vi "packageTelemetrySnapshot.vi"(8 "Error In":errorcluster, 10 "All Data":T2 {"Power Readings"."Current" format="%#.3g A"; "Power Readings"."Power" format="%#.3g W"; "Power Readings"."Shunt Voltage" format=" %#.3g V"; "Power Readings"."Bus Voltage" format="%#.3g V"; "Power Readings"."Voltage (Total)" format="%#.3g V"; "ThermalReadings"."Ambient Temp (°F)" format="%.2f °F"; "ThermalReadings"."Ambient Temp (°C)" format="%.2f °C"; "ThermalReadings"."Object Temp (°F)" format="%.2f °F"; "ThermalReadings"."Object Temp (°C)" format="%.2f °C"; "CPU loads"."ISR (%)" format="%#.2f"; "CPU loads"."Idle (%)" format="%#.2f"; "CPU loads"."Background (%)" format="%#.2f"; "CPU loads"."Normal (%)" format="%#.2f"; "CPU loads"."Above Normal (%)" format="%#.2f"; "CPU loads"."High (%)" format="%#.2f"; "CPU loads"."Timed Structures (%)" format="%#.2f"; "CPU loads"."Time Critical (%)" format="%#.2f"; "CPU loads"."Total (%)" format="%#.2f"}, 11 "Send Non-Critical Data":bool) -> (0 "Error Out":errorcluster, 2 "Pod Health":T1, 3 "Latest Critical Telemetry":T12)   [LabVIEW 2018]
uses:
  Type Defs/PodState.ctl
  Type Defs/criticalTelemetry.ctl
  Type Defs/prettyTelemetry.ctl
  Type Defs/ThermalReadings.ctl
  Type Defs/PodHealthConfig.ctl
  Sensors/Power Sensor - Adafruit INA219/INA219 Measurements.ctl
  Type Defs/tempReadings.ctl
  Type Defs/AnalogPressureReading.ctl
  Type Defs/allLaserReadings.ctl
  Type Defs/tofReading.ctl
  <vilib>/Utility/RT CPU Load.ctl
  Type Defs/pressureReading.ctl
  Type Defs/allData.ctl
  Type Defs/laserReading.ctl
  Type Defs/PodHealth.ctl
panel:
  out "UDP Data Packet":string
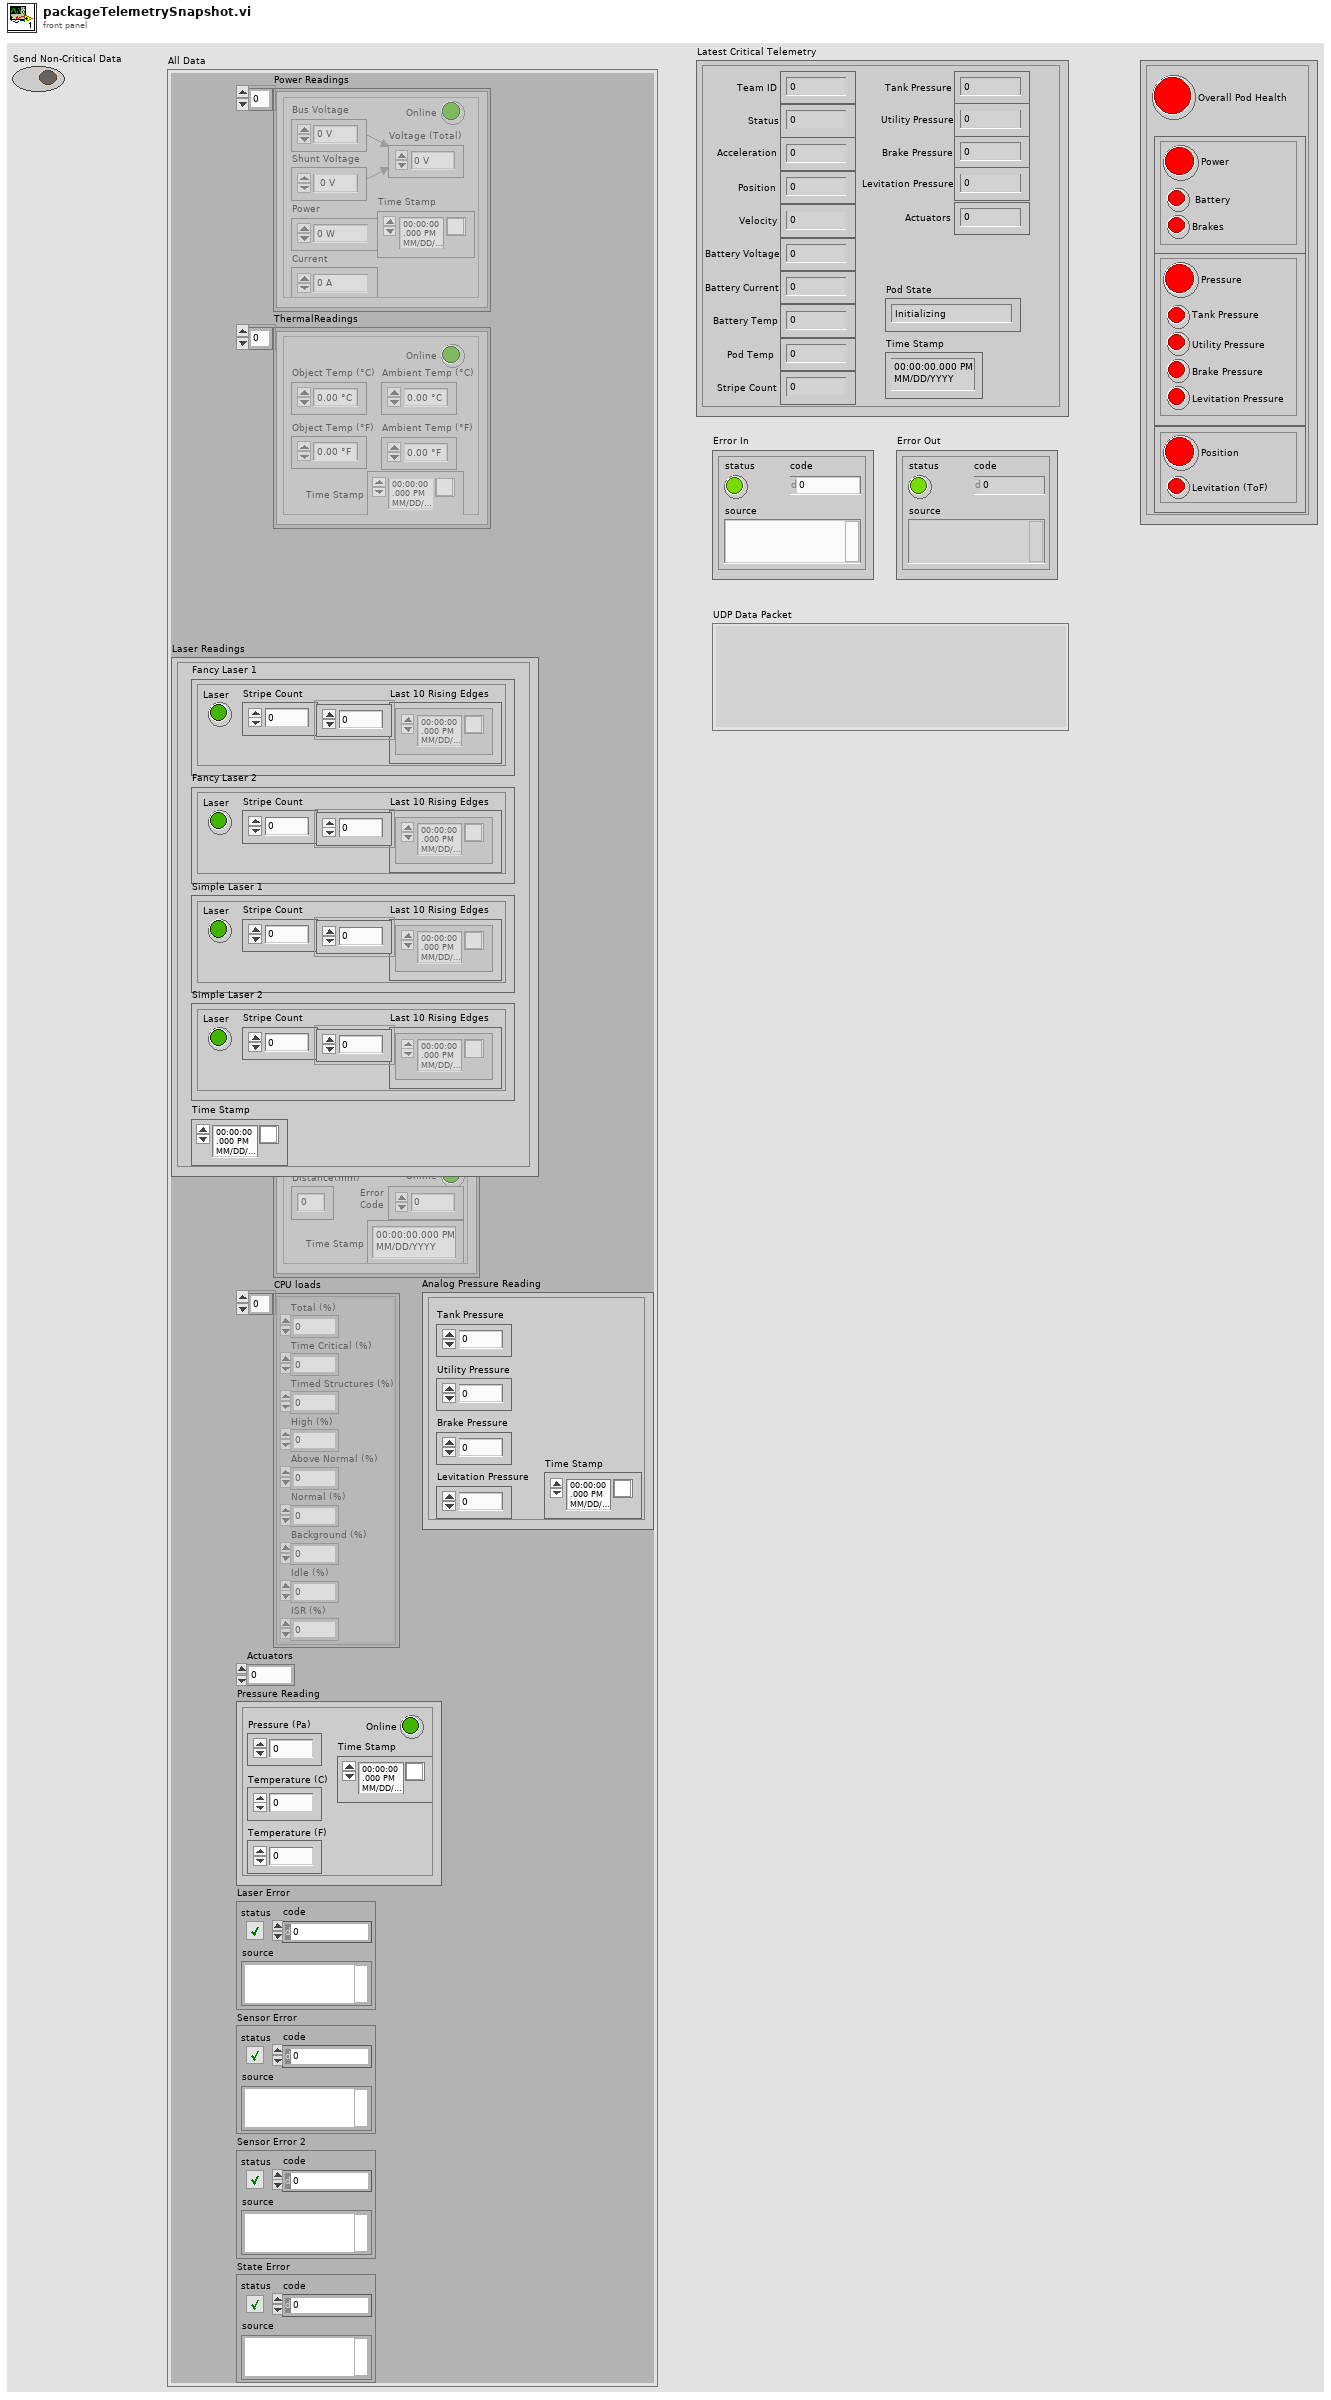
[diagram p1: front panel]
types:
  T1 = typedef "PodHealth.ctl" = cluster{"Overall Pod Health":bool, "Power":cluster{"Power":bool, " Battery":bool, "Brakes":bool}, "Pressure":cluster{"Pressure":bool, "Tank Pressure":bool, "Utility Pressure":bool, "Brake Pressure":bool, "Levitation Pressure":bool}, "Position":cluster{"Position":bool, "Levitation (ToF)":bool}}
  T2 = typedef "allData.ctl" = cluster{"Power Readings":T3[], "ThermalReadings":T4[], "Analog Pressure Reading":T5, "Laser Readings":T6, "Pod State":T8, "seconds since 1Jan1904":timestamp, "ToF Readings":T9[], "CPU loads":T10[], "Actuators":u32, "Pressure Reading":T11, "Laser Error":errorcluster, "Sensor Error":errorcluster, "Sensor Error 2":errorcluster, "State Error":errorcluster}
  T3 = typedef "INA219 Measurements.ctl" = cluster{"Voltage (Total)":dbl, "Bus Voltage":dbl, "Shunt Voltage":dbl, "Power":dbl, "Current":dbl, "Online":bool, "Time Stamp":timestamp}
  T4 = typedef "tempReadings.ctl" = cluster{"Object Temp (°C)":dbl, "Object Temp (°F)":dbl, "Ambient Temp (°C)":dbl, "Ambient Temp (°F)":dbl, "Online":bool, "Time Stamp":timestamp}
  T5 = typedef "AnalogPressureReading.ctl" = cluster{"Tank Pressure":dbl, "Utility Pressure":dbl, "Brake Pressure":dbl, "Levitation Pressure":dbl, "Time Stamp":timestamp}
  T6 = typedef "allLaserReadings.ctl" = cluster{"Fancy Laser 1":T7, "Fancy Laser 2":T7, "Simple Laser 1":T7, "Simple Laser 2":T7, "Time Stamp":timestamp}
  T7 = typedef "laserReading.ctl" = cluster{"Laser":bool, "Stripe Count":u32, "Last 10 Rising Edges":timestamp[]}
  T8 = typedef "PodState.ctl" = enum16{"Initializing", "Pre-flight Testing", "Ready", "Pushing", "Coast", "Braking", "Pod-Stop", "Fault"}
  T9 = typedef "tofReading.ctl" = cluster{"Distance(mm)":u8, "Online":bool, "Error\nCode":u8, "Time Stamp":timestamp}
  T10 = typedef "NI_Real-Time Target Support.lvlib/RT CPU Load.ctl" = cluster{"Total (%)":dbl, "Time Critical (%)":dbl, "Timed Structures (%)":dbl, "High (%)":dbl, "Above Normal (%)":dbl, "Normal (%)":dbl, "Background (%)":dbl, "Idle (%)":dbl, "ISR (%)":dbl}
  T11 = typedef "pressureReading.ctl" = cluster{"Time Stamp":timestamp, "Online":bool, "Temperature (C)":dbl, "Pressure (Pa)":dbl, "Temperature (F)":dbl}
  T12 = typedef "criticalTelemetry.ctl" = cluster{"Team ID":u8, "Status":u8, "Acceleration":dbl, "Position":dbl, "Velocity":dbl, "Battery Voltage":dbl, "Battery Current":dbl, "Battery Temp":dbl, "Pod Temp":dbl, "Stripe Count":u32, "Tank Pressure":dbl, "Utility Pressure":dbl, "Brake Pressure":dbl, "Actuators":u32, "Pod State":T8, "Time Stamp":timestamp, "Levitation Pressure":dbl}
  T13 = typedef "prettyTelemetry.ctl" = cluster{"Battery Current (A)":dbl, "Brake Current (A)":dbl, "Battery Voltage (V)":dbl, "Brake Voltage (V)":dbl, "Tank Pressure (PSI)":dbl, "Utility Pressure (PSI)":dbl, "Levitation Pressure (PSI)":dbl, "Brake Pressure (PSI)":dbl, "ToF 1 (mm)":dbl, "ToF 2 (mm)":dbl, "ToF 3 (mm)":dbl, "ToF 4 (mm)":dbl, "Maglock 1 (mm)":dbl, "Maglock 2 (mm)":dbl, "Maglock 3 (mm)":dbl, "Maglock 4 (mm)":dbl}
  T14 = typedef "positionData.ctl" = cluster{"Position (m)":dbl, "Velocity (m/s)":dbl, "Acceleration (m/s^2)":dbl}
  T15 = typedef "ThermalReadings.ctl" = cluster{"Temp1":dbl, "Temp2":dbl, "Temp3":dbl, "Temp4":dbl}
  T16 = typedef "PodHealthConfig.ctl" = cluster{"Power":cluster{"Batt. Current Max (A)":dbl, " Batt. Current Min (A)":dbl, "Batt. Voltage Min (V)":dbl, "Batt. Voltage Max (V)":dbl, "Brake Current Max (A)":dbl, " Brake Current Min (A)":dbl, "Brake Voltage Min (V)":dbl, "Brake Voltage Max (V)":dbl}, "Pressure":cluster{"Tank Max (PSI)":dbl, "Tank Min (PSI)":dbl, "Utility Max (PSI)":dbl, "Utility Min (PSI)":dbl, "Brake Max (PSI)":dbl, "Brake Min (PSI)":dbl, "Levitation Max (PSI)":dbl, "Levitation Min (PSI)":dbl}, "Position":cluster{"Lev. Min (mm)":dbl, "Lev. Max (mm)":dbl}}
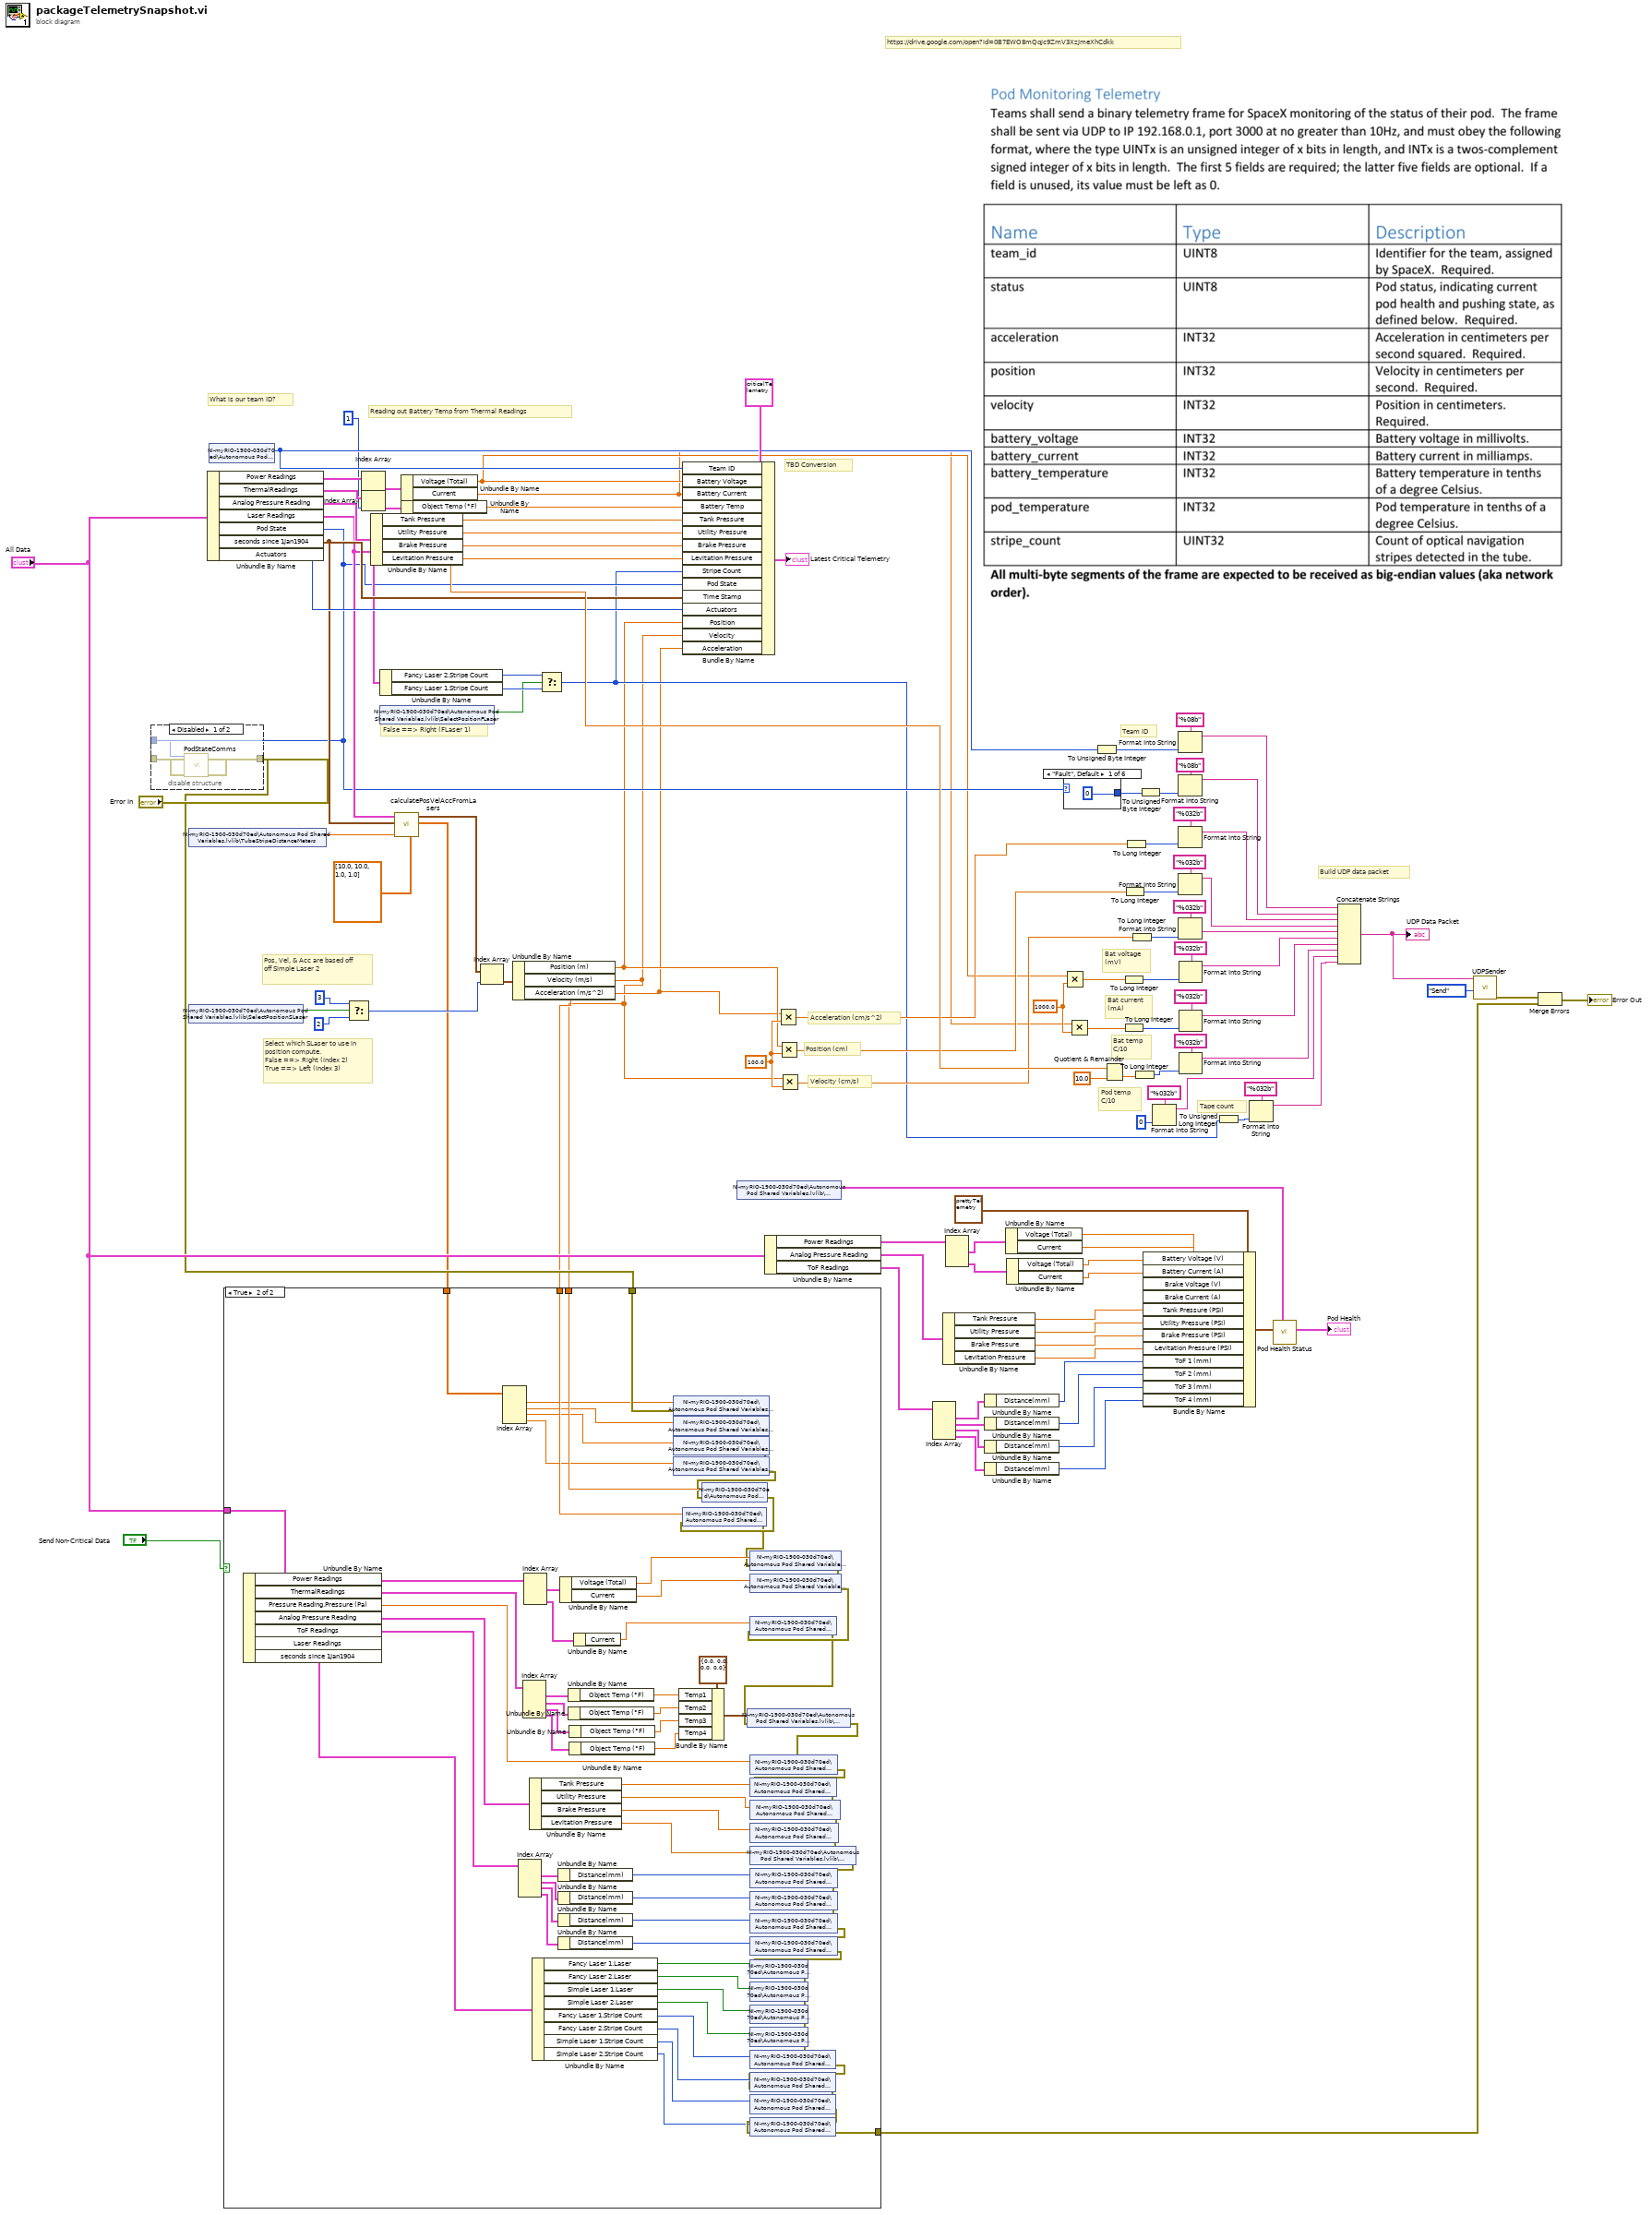
[diagram p0: block diagram]
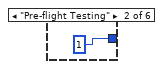
[diagram p2: hidden frame]
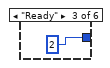
[diagram p3: hidden frame]
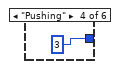
[diagram p4: hidden frame]
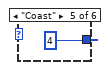
[diagram p5: hidden frame]
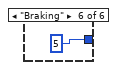
[diagram p6: hidden frame]
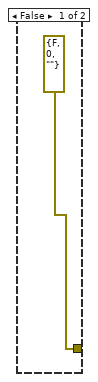
[diagram p8: hidden frame]
diagram:
  w57 = 100.0 ("32bit integer")
  w67 = 1000.0 ("32bit integer")
  # "Reading out Battery Temp from Thermal Readings"
  # "Position (cm)"
  # "Velocity (cm/s)"
  # "Acceleration (cm/s^2)"
  # "False ==> RIght (FLaser 1)"
  # "Pod temp\nC/10"
  # "Tape count"
  # "Team ID"
  # "Bat temp\nC/10"
  # "Bat current\n(mA)"
  # "Bat voltage\n(mV)"
  # "Build UDP data packet"
  # "Select which SLaser to use in position compute.\nFalse ==> Right (index 2)\nTrue ==> Left (index 3)"
  # "Pos, Vel, & Acc are based off off Simple Laser 2"
  # "What is our team ID?"
  # "https://drive.google.com/open?id=0B7EWO8mQqjc9ZmV3XzJmeXhCdkk"
  # "TBD Conversion"
  n1 = shared-variable "NI-myRIO-1900-030d70ed\\Autonomous Pod Shared Variables.lvlib\\TubeStripeDistanceMeters"() -> (w87:dbl)  [unwired: 1 in, 1 out]
  n2 = shared-variable "NI-myRIO-1900-030d70ed\\Autonomous Pod Shared Variables.lvlib\\SelectPositionSLaser"() -> (w92:bool)  [unwired: 1 in, 1 out]
  n3 = Unbundle By Name("All Data") -> ("Power Readings"=w110:T3[], "ThermalReadings"=w107:T4[], "Analog Pressure Reading"=w104:T5, "Laser Readings"=w95:T6, "Pod State"=w68:T8, "seconds since 1Jan1904"=w96:timestamp, "Actuators"=w98:u32)
  n4 = disable-structure shown="Disabled" {
    disable-tunnel: w68 -> [w113 _]
    disable-tunnel: "Error In" -> [w112 w114]
    disable-tunnel: [w111 w114] -> w7
    frame Disabled {
      n5 = call "PodStateComms.vi"("error in"=w112, "Pod State"=w113) -> ("error out"=w111:errorcluster)  [unwired: 9 in]
    }
    frame Enabled {
    }
  }
  n6 = shared-variable "NI-myRIO-1900-030d70ed\\Autonomous Pod Shared Variables.lvlib\\TeamID"() -> (w62:u8)  [unwired: 1 in, 1 out]
  n7 = Select(t=3 ("index"), s=w92, f=2 ("index")) -> (s? t:f=w89:i32)
  n8 = Index Array(array=w110) -> (element=w108:T3)  [unwired: 1 in]
  n9 = Index Array(array=w107, index=1) -> (element=w106:T4)
  n10 = Unbundle By Name(w104) -> ("Tank Pressure"=w103:dbl, "Utility Pressure"=w102:dbl, "Brake Pressure"=w101:dbl, "Levitation Pressure"=w41:dbl)
  n11 = Unbundle By Name(w95) -> ("Fancy Laser 2.Stripe Count"=w65:u32, "Fancy Laser 1.Stripe Count"=w64:u32)
  n12 = shared-variable "NI-myRIO-1900-030d70ed\\Autonomous Pod Shared Variables.lvlib\\SelectPositionFLaser"() -> (w63:bool)  [unwired: 1 in, 1 out]
  n13 = call "calculatePosVelAccFromLasers.vi"("Velocity Timeouts"=dbl[] [10.0, 10.0, 1.0, 1.0], "Distance between Tube Stripes"=w87, "Right Now"=w96, "Laser Readings"=w95) -> ("Positions"=w4:dbl[], "Position Calculations"=w93:T14[])  [unwired: 6 in]
  n14 = Unbundle By Name(w108) -> ("Voltage (Total)"=w14:dbl, "Current"=w13:dbl)
  n15 = Unbundle By Name(w106) -> ("Object Temp (°F)"=w105:dbl)
  n16 = Index Array(array=w93, index=w89) -> (element=w94:T14)
  n17 = Unbundle By Name(w94) -> ("Position (m)"=w8:dbl, "Velocity (m/s)"=w5:dbl, "Acceleration (m/s^2)"=w6:dbl)
  n18 = case shown="True" "Send Non-Critical Data" {
    tunnel: "All Data" -> [_ w188]
    tunnel: [errorcluster {"status"=FALSE, "code"=0, "source"=""} ("error IO") w145] -> w44
    tunnel: w7 -> [_ w144]
    tunnel: w6 -> [_ w143]
    tunnel: w5 -> [_ w142]
    tunnel: w4 -> [_ w135]
    frame False {
    }
    frame True {
      n19 = Unbundle By Name(w188) -> ("Power Readings"=w189:T3[], "ThermalReadings"=w191:T4[], "Pressure Reading.Pressure (Pa)"=w185:dbl, "Analog Pressure Reading"=w192:T5, "ToF Readings"=w180:T9[], "Laser Readings"=w171:T6)  [unwired: 1 out]
      n20 = Index Array(array=w135) -> (element #1=w134:dbl, element #2=w133:dbl, element #3=w132:dbl, element #4=w131:dbl)  [unwired: 4 in]
      n21 = Index Array(array=w180) -> (element #1=w179:T9, element #2=w172:T9, element #3=w173:T9, element #4=w174:T9)  [unwired: 4 in]
      n22 = Index Array(array=w191) -> (element #1=w127:T4, element #2=w126:T4, element #3=w125:T4, element #4=w124:T4)  [unwired: 4 in]
      n23 = Index Array(array=w189) -> (element #1=w190:T3, element #3=w119:T3)  [unwired: 3 in, 1 out]
      n24 = Unbundle By Name(w192) -> ("Tank Pressure"=w184:dbl, "Utility Pressure"=w183:dbl, "Brake Pressure"=w182:dbl, "Levitation Pressure"=w181:dbl)
      n25 = Unbundle By Name(w171) -> ("Fancy Laser 1.Laser"=w170:bool, "Fancy Laser 2.Laser"=w169:bool, "Simple Laser 1.Laser"=w168:bool, "Simple Laser 2.Laser"=w167:bool, "Fancy Laser 1.Stripe Count"=w166:u32, "Fancy Laser 2.Stripe Count"=w165:u32, "Simple Laser 1.Stripe Count"=w147:u32, "Simple Laser 2.Stripe Count"=w146:u32)
      n26 = Unbundle By Name(w179) -> ("Distance(mm)"=w178:u8)
      n27 = Unbundle By Name(w172) -> ("Distance(mm)"=w175:u8)
      n28 = Unbundle By Name(w173) -> ("Distance(mm)"=w176:u8)
      n29 = Unbundle By Name(w174) -> ("Distance(mm)"=w177:u8)
      n30 = Unbundle By Name(w190) -> ("Voltage (Total)"=w187:dbl, "Current"=w186:dbl)
      n31 = Unbundle By Name(w127) -> ("Object Temp (°F)"=w123:dbl)
      n32 = Unbundle By Name(w126) -> ("Object Temp (°F)"=w122:dbl)
      n33 = Unbundle By Name(w125) -> ("Object Temp (°F)"=w121:dbl)
      n34 = Unbundle By Name(w124) -> ("Object Temp (°F)"=w120:dbl)
      n35 = Unbundle By Name(w119) -> ("Current"=w118:dbl)
      n36 = shared-variable "NI-myRIO-1900-030d70ed\\Autonomous Pod Shared Variables.lvlib\\PositionFLaser1"(w134, error in=w144) -> (error out=w141:errorcluster)
      n37 = shared-variable "NI-myRIO-1900-030d70ed\\Autonomous Pod Shared Variables.lvlib\\PositionFLaser2"(w133, error in=w141) -> (error out=w140:errorcluster)
      n38 = shared-variable "NI-myRIO-1900-030d70ed\\Autonomous Pod Shared Variables.lvlib\\PositionSLaser1"(w132, error in=w140) -> (error out=w139:errorcluster)
      n39 = shared-variable "NI-myRIO-1900-030d70ed\\Autonomous Pod Shared Variables.lvlib\\PositionSLaser2"(w131, error in=w139) -> (error out=w138:errorcluster)
      n40 = Bundle By Name(cluster=T15 {"Temp1"=0.0, "Temp2"=0.0, "Temp3"=0.0, "Temp4"=0.0}, "Temp1"=w123, "Temp2"=w122, "Temp3"=w121, "Temp4"=w120) -> (w129:T15)
      n41 = shared-variable "NI-myRIO-1900-030d70ed\\Autonomous Pod Shared Variables.lvlib\\Velocity"(w142, error in=w138) -> (error out=w137:errorcluster)
      n42 = shared-variable "NI-myRIO-1900-030d70ed\\Autonomous Pod Shared Variables.lvlib\\Acceleration"(w143, error in=w137) -> (error out=w136:errorcluster)
      n43 = shared-variable "NI-myRIO-1900-030d70ed\\Autonomous Pod Shared Variables.lvlib\\BatteryVoltage"(w187, error in=w136) -> (error out=w164:errorcluster)
      n44 = shared-variable "NI-myRIO-1900-030d70ed\\Autonomous Pod Shared Variables.lvlib\\BatteryCurrent"(w186, error in=w164) -> (error out=w117:errorcluster)
      n45 = shared-variable "NI-myRIO-1900-030d70ed\\Autonomous Pod Shared Variables.lvlib\\BrakeCurrent"(w118, error in=w117) -> (error out=w116:errorcluster)
      n46 = shared-variable "NI-myRIO-1900-030d70ed\\Autonomous Pod Shared Variables.lvlib\\ThermalReadings"(w129, error in=w116) -> (error out=w128:errorcluster)
      n47 = shared-variable "NI-myRIO-1900-030d70ed\\Autonomous Pod Shared Variables.lvlib\\TubePressure"(w185, error in=w128) -> (error out=w163:errorcluster)
      n48 = shared-variable "NI-myRIO-1900-030d70ed\\Autonomous Pod Shared Variables.lvlib\\HighPressure"(w184, error in=w163) -> (error out=w162:errorcluster)
      n49 = shared-variable "NI-myRIO-1900-030d70ed\\Autonomous Pod Shared Variables.lvlib\\UtilityPressure"(w183, error in=w162) -> (error out=w161:errorcluster)
      n50 = shared-variable "NI-myRIO-1900-030d70ed\\Autonomous Pod Shared Variables.lvlib\\BrakePressure"(w182, error in=w161) -> (error out=w160:errorcluster)
      n51 = shared-variable "NI-myRIO-1900-030d70ed\\Autonomous Pod Shared Variables.lvlib\\LevitationPressure"(w181, error in=w160) -> (error out=w159:errorcluster)
      n52 = shared-variable "NI-myRIO-1900-030d70ed\\Autonomous Pod Shared Variables.lvlib\\ToF1Distance"(w178, error in=w159) -> (error out=w158:errorcluster)
      n53 = shared-variable "NI-myRIO-1900-030d70ed\\Autonomous Pod Shared Variables.lvlib\\ToF2Distance"(w175, error in=w158) -> (error out=w157:errorcluster)
      n54 = shared-variable "NI-myRIO-1900-030d70ed\\Autonomous Pod Shared Variables.lvlib\\ToF3Distance"(w176, error in=w157) -> (error out=w156:errorcluster)
      n55 = shared-variable "NI-myRIO-1900-030d70ed\\Autonomous Pod Shared Variables.lvlib\\ToF4Distance"(w177, error in=w156) -> (error out=w155:errorcluster)
      n56 = shared-variable "NI-myRIO-1900-030d70ed\\Autonomous Pod Shared Variables.lvlib\\Laser1"(w170, error in=w155) -> (error out=w154:errorcluster)
      n57 = shared-variable "NI-myRIO-1900-030d70ed\\Autonomous Pod Shared Variables.lvlib\\Laser2"(w169, error in=w154) -> (error out=w153:errorcluster)
      n58 = shared-variable "NI-myRIO-1900-030d70ed\\Autonomous Pod Shared Variables.lvlib\\Laser3"(w168, error in=w153) -> (error out=w152:errorcluster)
      n59 = shared-variable "NI-myRIO-1900-030d70ed\\Autonomous Pod Shared Variables.lvlib\\Laser4"(w167, error in=w152) -> (error out=w151:errorcluster)
      n60 = shared-variable "NI-myRIO-1900-030d70ed\\Autonomous Pod Shared Variables.lvlib\\StripeCount1"(w166, error in=w151) -> (error out=w150:errorcluster)
      n61 = shared-variable "NI-myRIO-1900-030d70ed\\Autonomous Pod Shared Variables.lvlib\\StripeCount2"(w165, error in=w150) -> (error out=w149:errorcluster)
      n62 = shared-variable "NI-myRIO-1900-030d70ed\\Autonomous Pod Shared Variables.lvlib\\StripeCount3"(w147, error in=w149) -> (error out=w148:errorcluster)
      n63 = shared-variable "NI-myRIO-1900-030d70ed\\Autonomous Pod Shared Variables.lvlib\\StripeCount4"(w146, error in=w148) -> (error out=w145:errorcluster)
    }
  }
  n64 = Select(t=w65, s=w63, f=w64) -> (s? t:f=w42:u32)
  n65 = Bundle By Name(cluster=T12 {"Team ID"=0, "Status"=0, "Acceleration"=0.0, "Position"=0.0, "Velocity"=0.0, "Battery Voltage"=0.0, "Battery Current"=0.0, "Battery Temp"=0.0, "Pod Temp"=0.0, "Stripe Count"=0, "Tank Pressure"=0.0, "Utility Pressure"=0.0, "Brake Pressure"=0.0, "Actuators"=0, "Pod State"=enum."Initializing", "Time Stamp"=timestamp(0 s since 1904-01-01), "Levitation Pressure"=0.0} ("Latest Critical Telemetry"), "Team ID"=w62, "Battery Voltage"=w14, "Battery Current"=w13, "Battery Temp"=w105, "Tank Pressure"=w103, "Utility Pressure"=w102, "Brake Pressure"=w101, "Levitation Pressure"=w41, "Stripe Count"=w42, "Pod State"=w68, "Time Stamp"=w96, "Actuators"=w98, "Position"=w8, "Velocity"=w5, "Acceleration"=w6) -> (→"Latest Critical Telemetry":T12)
  n66 = shared-variable "NI-myRIO-1900-030d70ed\\Autonomous Pod Shared Variables.lvlib\\PodHealthConfig"() -> (w15:T16)  [unwired: 1 in, 1 out]
  n67 = Unbundle By Name("All Data") -> ("Power Readings"=w24:T3[], "Analog Pressure Reading"=w34:T5, "ToF Readings"=w29:T9[])
  n68 = Multiply(x=w6, y=w57) -> (x*y=w59:dbl)
  n69 = Multiply(x=w8, y=w57) -> (x*y=w55:dbl)
  n70 = Multiply(x=w5, y=w57) -> (x*y=w58:dbl)
  n71 = Index Array(array=w29) -> (element #1=w30:T9, element #2=w33:T9, element #3=w32:T9, element #4=w31:T9)  [unwired: 4 in]
  n72 = Unbundle By Name(w34) -> ("Tank Pressure"=w38:dbl, "Utility Pressure"=w37:dbl, "Brake Pressure"=w35:dbl, "Levitation Pressure"=w36:dbl)
  n73 = Index Array(array=w24) -> (element #1=w23:T3, element #3=w22:T3)  [unwired: 3 in, 1 out]
  n74 = Unbundle By Name(w30) -> ("Distance(mm)"=w28:u8)
  n75 = Unbundle By Name(w33) -> ("Distance(mm)"=w27:u8)
  n76 = Unbundle By Name(w32) -> ("Distance(mm)"=w26:u8)
  n77 = Unbundle By Name(w31) -> ("Distance(mm)"=w25:u8)
  n78 = Unbundle By Name(w23) -> ("Voltage (Total)"=w21:dbl, "Current"=w20:dbl)
  n79 = Unbundle By Name(w22) -> ("Voltage (Total)"=w19:dbl, "Current"=w18:dbl)
  n80 = Multiply(x=w14, y=w67) -> (x*y=w12:dbl)
  n81 = case shown="\"Fault\", Default" w68 {
    tunnel: [u8 0 ("number") u8 1 ("number") u8 2 ("number") u8 3 ("number") u8 4 ("number") u8 5 ("number")] -> w82
    frame "Fault", Default {
    }
    frame "Pre-flight Testing" {
    }
    frame "Ready" {
    }
    frame "Pushing" {
    }
    frame "Coast" {
    }
    frame "Braking" {
    }
  }
  n82 = Multiply(x=w13, y=w67) -> (x*y=w10:dbl)
  n83 = To Unsigned Byte Integer(number=w62) -> (unsigned 8bit integer=w85:u8)
  n84 = Quotient & Remainder(x=w105, y=10.0 ("32bit integer")) -> (floor(x/y)=w3:dbl)  [unwired: 1 out]
  n85 = To Long Integer(number=w12) -> (32bit integer=w11:i32)
  n86 = To Long Integer(number=w10) -> (32bit integer=w9:i32)
  n87 = To Long Integer(number=w55) -> (32bit integer=w56:i32)
  n88 = To Long Integer(number=w59) -> (32bit integer=w60:i32)
  n89 = To Long Integer(number=w58) -> (32bit integer=w61:i32)
  n90 = To Long Integer(number=w3) -> (32bit integer=w2:i32)
  n91 = To Unsigned Byte Integer(number=w82) -> (unsigned 8bit integer=w83:u8)
  n92 = Bundle By Name(cluster=T13 {"Battery Current (A)"=0.0, "Brake Current (A)"=0.0, "Battery Voltage (V)"=0.0, "Brake Voltage (V)"=0.0, "Tank Pressure (PSI)"=0.0, "Utility Pressure (PSI)"=0.0, "Levitation Pressure (PSI)"=0.0, "Brake Pressure (PSI)"=0.0, "ToF 1 (mm)"=0.0, "ToF 2 (mm)"=0.0, "ToF 3 (mm)"=0.0, "ToF 4 (mm)"=0.0, "Maglock 1 (mm)"=0.0, "Maglock 2 (mm)"=0.0, "Maglock 3 (mm)"=0.0, "Maglock 4 (mm)"=0.0} ("Telemetry"), "Battery Voltage (V)"=w21, "Battery Current (A)"=w20, "Brake Voltage (V)"=w19, "Brake Current (A)"=w18, "Tank Pressure (PSI)"=w38, "Utility Pressure (PSI)"=w37, "Brake Pressure (PSI)"=w35, "Levitation Pressure (PSI)"=w36, "ToF 1 (mm)"=w28, "ToF 2 (mm)"=w27, "ToF 3 (mm)"=w26, "ToF 4 (mm)"=w25) -> (w17:T13)
  n93 = Format Into String(format string="%032b", 0 ("input 1")) -> (resulting string=w54:string)  [unwired: 2 in, 1 out]
  n94 = Format Into String(format string="%08b", w85) -> (resulting string=w73:string)  [unwired: 2 in, 1 out]
  n95 = Format Into String(format string="%08b", w83) -> (resulting string=w72:string)  [unwired: 2 in, 1 out]
  n96 = Format Into String(format string="%032b", w60) -> (resulting string=w71:string)  [unwired: 2 in, 1 out]
  n97 = Format Into String(format string="%032b", w56) -> (resulting string=w49:string)  [unwired: 2 in, 1 out]
  n98 = Format Into String(format string="%032b", w61) -> (resulting string=w50:string)  [unwired: 2 in, 1 out]
  n99 = Format Into String(format string="%032b", w11) -> (resulting string=w51:string)  [unwired: 2 in, 1 out]
  n100 = Format Into String(format string="%032b", w9) -> (resulting string=w52:string)  [unwired: 2 in, 1 out]
  n101 = Format Into String(format string="%032b", w2) -> (resulting string=w53:string)  [unwired: 2 in, 1 out]
  n102 = To Unsigned Long Integer(number=w42) -> (unsigned 32bit integer=w74:u32)
  n103 = Format Into String(format string="%032b", w74) -> (resulting string=w45:string)  [unwired: 2 in, 1 out]
  n104 = call "Pod Health Status.vi"("Pod Health Configuration"=w15, "Telemetry"=w17) -> ("Pod Health"=→"Pod Health":T1)  [unwired: 9 in]
  n105 = Concatenate Strings(w73, w72, w71, w49, w50, w51, w52, w53, w54, w45) -> (w48:string)
  "UDP Data Packet" <- w48
  n106 = call "UDPSender.vi"("Action"=enum16{"Send", "Initialize", "Close"}."Send", "Pod Monitoring Telemetry"=w48) -> ("error out"=w46:errorcluster)  [unwired: 9 in]
  n107 = Merge Errors(w46, w44) -> (→"Error Out":errorcluster)
